vi "My Grayscale Wiener Filter.vi"() -> ()   [LabVIEW 2017]
doc: "This example showing the use case of Wiener Filter in imageprocessing. Wiener filter is a method of restoring image in the presence of blur (and noise) in the case when the blur kernel is known. In the given example I using Gaussian blur. This algorithm also can be used from restoring “motion blurred” images.\n\nA blurred or degraded image can be approximately described by equation Dst(x,y) = PSF * Src(x,y), where Src and Dst are source and result images and PSF is distortion operator called Point Spread Function. The Wiener filter can be understood better in the frequency domain. For deconvolution we will perform Fourier Transform of the blurred image, then perform convolution with inversed PSF function, and after inverse Fourier transform we will get the original image. When you know the exact PSF, the results of deblurring can be really effective."
uses:
  <vilib>/Analysis/2dsp.llb/2D Real FFT.vi
  <vilib>/Analysis/2dsp.llb/2D Inverse Complex FFT.vi
  <vilib>/Analysis/2dsp.llb/2D Inverse Real FFT.vi
  <vilib>/Analysis/NI_AALPro.lvlib
panel:
  out "Recontstruction 2":dbl[][](graph)
  out "Recontstruction":dbl[][](graph)
  out "Original image":dbl[][](graph)
  in  "path to PNG file":path
  out "8-bit pixmap of loaded Image":i32[][](array[numeric])
  out "image from file":picture
  out "path":path
  in  "Sigma":dbl=3.0 min=1.0 max=3.0 step=0.1 format="%_3g"
  out "Blurred Image":u8[][](graph)
  # "Overview: This example showing the use case of Wiener Filter in image processing. Wiener filter is a method of restoring image in the presence of blur (and noise) in the case when the blur kernel is known. In the given example I using Gaussian blur. This algorithm also can be used from restoring “motion blurred” images."
  # "Wiener"
  # "Filter"
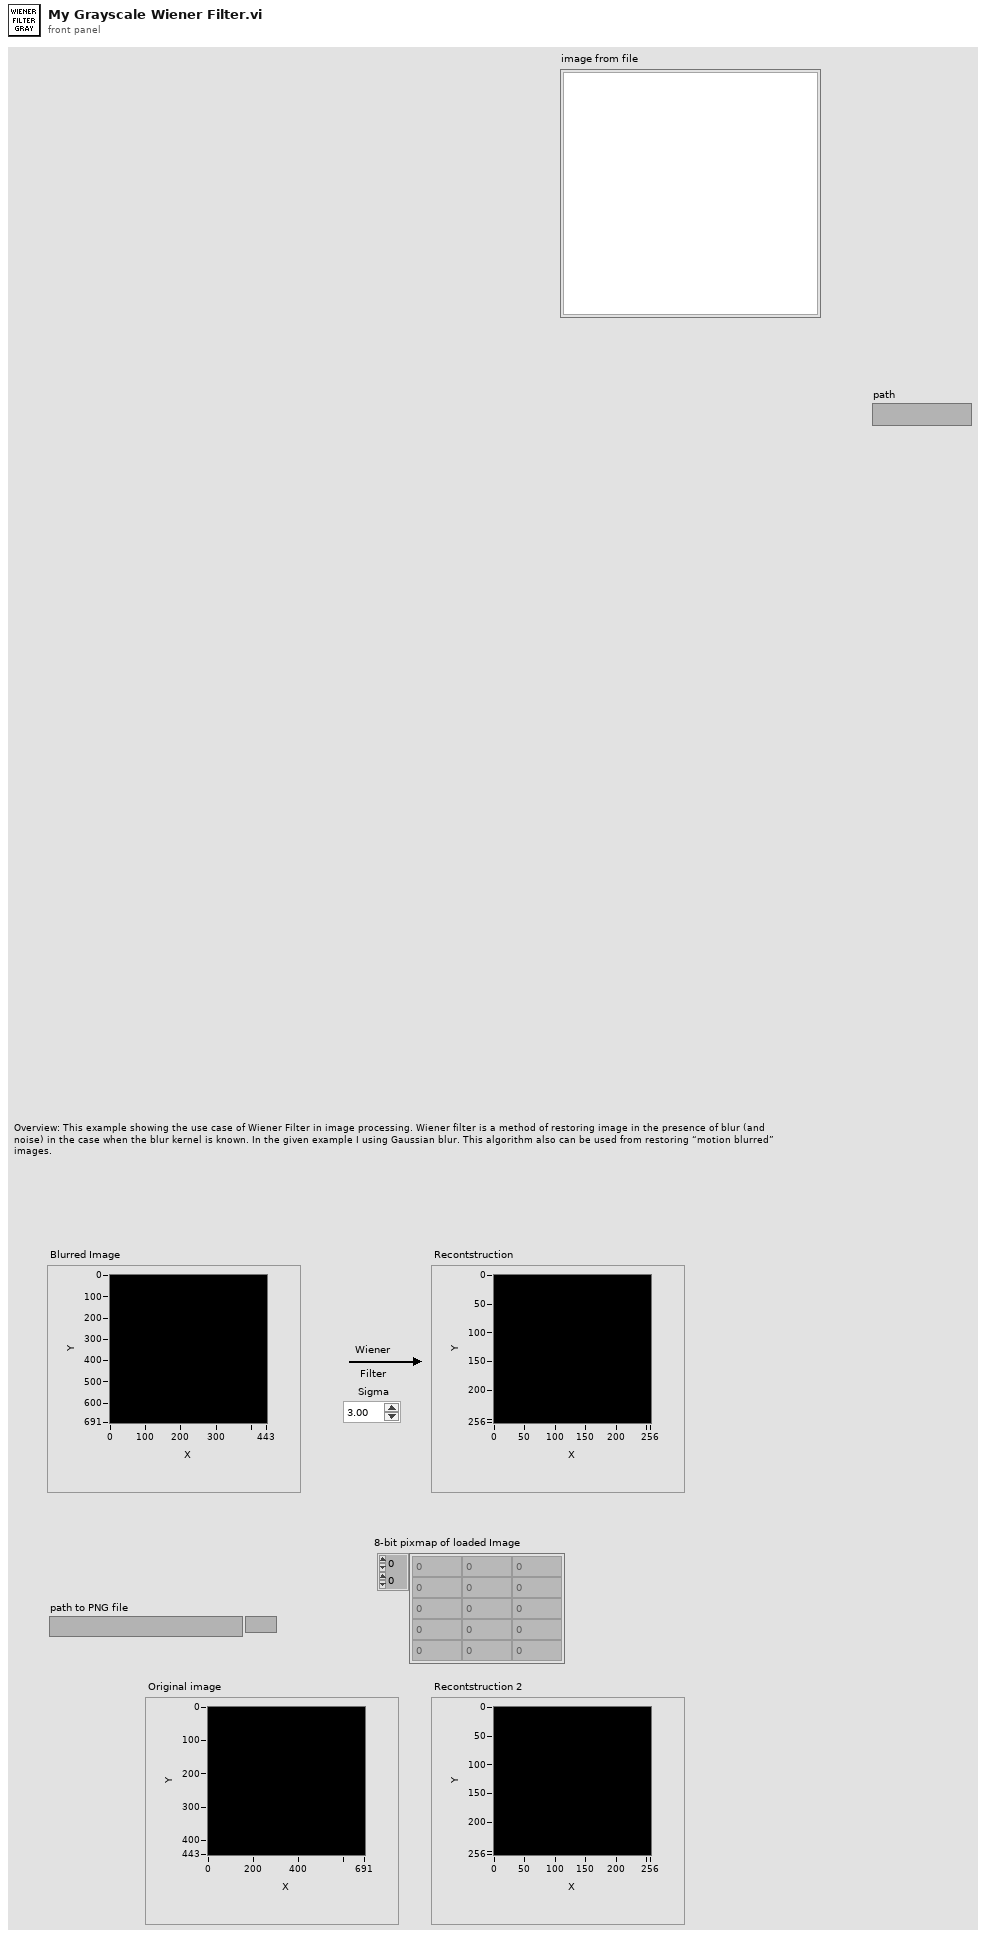
[diagram p1: front panel]
types:
  T1 = typedef "imagedata.ctl" = cluster{"image type":i32, "image depth":i32, "image":u8[], "mask":u8[], "colors":u32[], "Rectangle":cluster{"left":i16, "top":i16, "right":i16, "bottom":i16}}
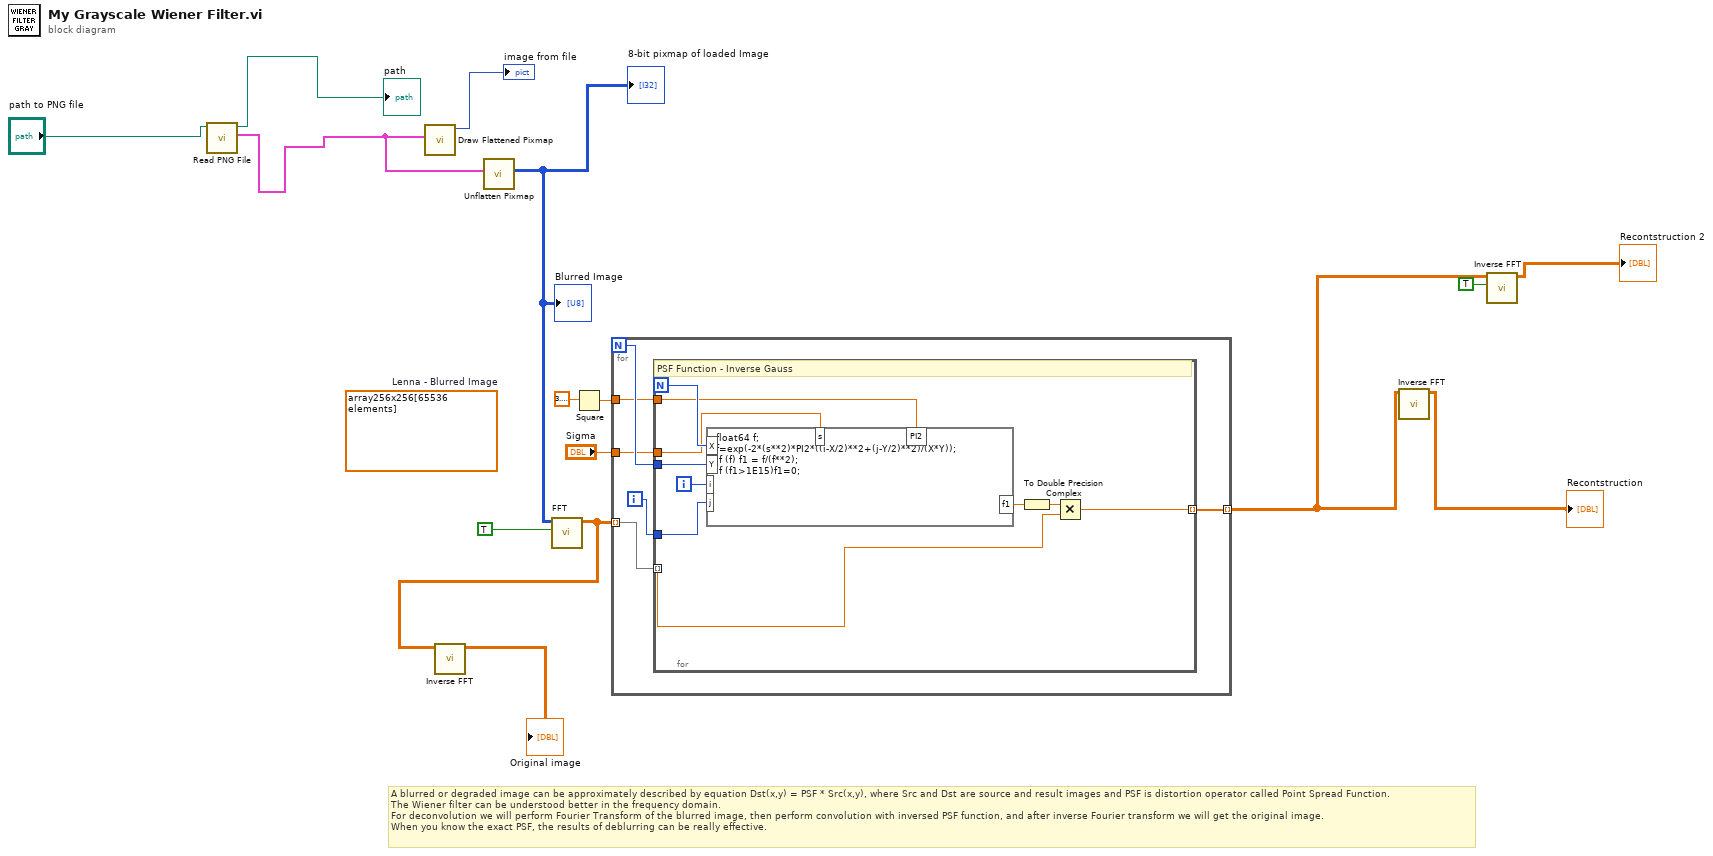
[diagram p0: block diagram]
diagram:
  (unwired) dbl[][] array256x256[65536 elements]  # Lenna - Blurred Image
  # "A blurred or degraded image can be approximately described by equation Dst(x,y) = PSF * Src(x,y), where Src and Dst are source and result images and PSF is distortion operator called Point Spread Function.\nThe Wiener filter can be understood better in the frequency domain.\nFor deconvolution we will perform Fourier Transform of the blurred image, then perform convolution with inversed PSF function, and after inverse Fourier transform we will get the original image.\nWhen you know the exact PSF, the results of deblurring can be really effective."
  n1 = call <vilib>:"Read PNG File.vi"("path to PNG file"="path to PNG file") -> ("image data"=w8:T1, "path"=→"path":path)  [unwired: 8 in, 1 out]
  n2 = call <vilib>:"Draw Flattened Pixmap.vi"("image data"=w8) -> ("new picture"=→"image from file":picture)  [unwired: 8 in]
  n3 = call <vilib>:"Unflatten Pixmap.vi"("image data"=w8) -> ("8-bit pixmap"=w1:u8[][])  [unwired: 4 in, 6 out]
  "Blurred Image" <- w1
  "8-bit pixmap of loaded Image" <- w1
  n4 = call-poly <vilib>:"FFT.vi"("shift?"=TRUE, "X"=w1) -> ("FFT {X}"=w7:cdb[][])  [unwired: 8 in, 1 out]
  n5 = call-poly <vilib>:"Inverse FFT.vi"("FFT {x}"=w7) -> ("X"=→"Original image":cdb[][])  [unwired: 9 in, 1 out]
  n6 = Square(x=3.141592653589793) -> (x^2=w13:dbl)
  n7 = for {
    N -> [w21]
    tunnel: w7 -> [w19] mode=indexing
    tunnel: [w18] -> w4 mode=indexing
    tunnel: w13 -> [w17]
    tunnel: "Sigma" -> [w16]
    i -> [w20]
    n8 = for {
      N -> [w31]
      tunnel: w21 -> [w30]
      tunnel: w20 -> [w28]
      tunnel: w19 -> [w22] mode=indexing
      tunnel: [w27] -> w18 mode=indexing
      tunnel: w17 -> [w24]
      tunnel: w16 -> [w23]
      i -> [w29]
      # "PSF Function - Inverse Gauss"
      n9 = formula code="float64 f;\nf=exp(-2*(s**2)*PI2*((i-X/2)**2+(j-Y/2)**2)/(X*Y));\nif (f) f1 = f/(f**2);\nif (f1>1E15)f1=0;"("s"=w23, "X"=w31, "i"=w29, "j"=w28, "PI2"=w24, "Y"=w30) -> ("f1"=w25:dbl)
      n10 = To Double Precision Complex(1:w25) -> (0:w26:cdb)
      n11 = Multiply(x=w26, y=w22) -> (x*y=w27:cdb)
    }
  }
  n12 = call-poly <vilib>:"Inverse FFT.vi"("FFT {X}"=w4) -> ("X"=→"Recontstruction":dbl[][])  [unwired: 9 in, 1 out]
  n13 = call-poly <vilib>:"Inverse FFT.vi"("shift?"=TRUE, "FFT {X}"=w4) -> ("X"=→"Recontstruction 2":dbl[][])  [unwired: 8 in, 1 out]
